vi "System Hidden Editor.vi"(6 "Channel":i32=1, 8 "Calibration in":string, 9 "Hardware in":string, 10 "Setup in":string, 11 "Editor seq info":T2 {"Steps config"."Loop Info"."unit scale" items=["Log", "Lin"]; "Steps config"."Loop Info"."unit dB ref" format="%#_6p"}) -> (1 "Step name out":string="Calibration Default", 2 "Setup out":string, 3 "Sequence channels & curves out":string[](array[string]))   [LabVIEW 2016]
uses:
  custom and Sc run Seq Sub VIs (x64).llb/editor seq info.ctl
  custom and Sc run Seq Sub VIs (x64).llb/Steps config.ctl
panel:
  in  "Wait for completion":bool
  in  "Working Directory":path
  in  "Command":string
  in  "custom setup cluster":T1={"Command Line"="", "Working Directory"=path "", "Wait for completion"=TRUE}
  in  "save":bool
  in  "cancel":bool
  # "Reminder: \nYou must edit this custom step from within a sequence for it to remember your settings."
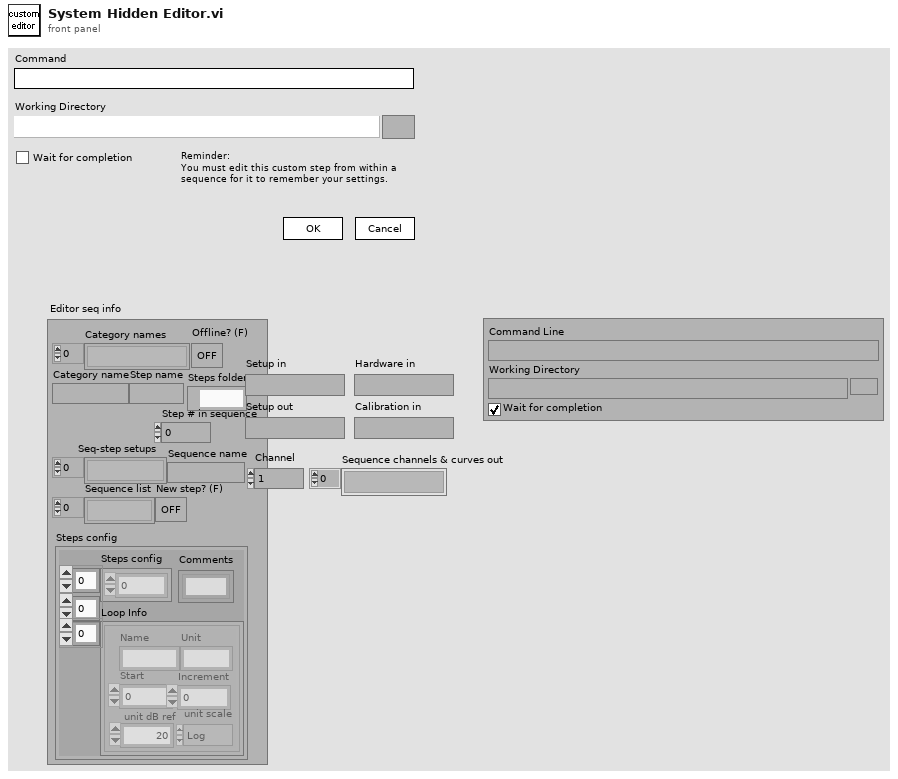
[diagram p1: front panel]
types:
  T1 = cluster{"Command Line":string, "Working Directory":path, "Wait for completion":bool}
  T2 = typedef "editor seq info.ctl" = cluster{"Category names":string[], "Category name":string, "Step name":string, "Step # in sequence":i32, "Seq-step setups":string[], "Sequence name":string, "Sequence list":string[], "New step? (F)":bool, "Steps config":T3, "Offline? (F)":bool, "Steps folder":path}
  T3 = typedef "Steps config.ctl" = cluster{"Steps config":i32[][], "Loop Info":cluster{"Name":string, "Start":dbl, "Increment":dbl, "Unit":string, "unit dB ref":dbl, "unit scale":u16}[], "Comments":string[]}
  T4 = typedef "seq step setup.ctl" = cluster{"Input Signal Channels":i32[], "Output Signal Channels":i32[], "Curves selected":string[][], "Curves generated":string[], "Step setup flat":string, "Trigger Signal Channel":i32, "Curves Generated Assumptions":cluster{"seq-setup in":string, "Relevant subset of mem list Grouping":cluster{T5[]}[]}}
  T5 = typedef "Memory List Grouping.ctl" = cluster{"item name":string, "parent":string, "Open?":bool, "Type":T6}
  T6 = typedef "Memory List Grouping - Item Type.ctl" = enum16{"item", "custom group", "auto group", "protected group"}
  T7 = typedef "waveform cluster.ctl" = cluster{"Name":string, "Waveform":cluster{"X0":dbl, "dX":dbl, "YDataRef":refnum<data-value>}, "X data":T8, "Y data":T8, "Y axis":T8, "X unit":string, "Y unit":string, "Y dB ref":dbl, "display Y":bool, "display X":bool, "Overload?":bool, "protected":bool, "Sqc history":string[], "Signal Channel ID":i32, "Plot Settings":cluster{"Color":u32, "Interpolation":u8, "Point Style":u8, "Line Style":u8, "Point Color":u32, "Line Width":u8, "Bar Plot Style":u8, "Fill To":i16}, "Test Info":string}
  T8 = typedef "Axis Unit Type.ctl" = u16
  T9 = typedef "data cluster.ctl" = cluster{"Name":string, "Curve":cluster{"x":dbl, "y":dbl, "z":dbl}[], "X data":T8, "Y data":T8, "Z data":T8, "X axis":u16, "Y axis":u16, "Z axis":u16, "X unit":string, "Y unit":string, "Z unit":string, "X dB ref":dbl, "Y dB ref":dbl, "Z dB ref":dbl, "single val":bool, "protected":bool, "display X":bool, "display Y":bool, "display Z":bool, "Plot Settings":cluster{"Color":u32, "Interpolation":u8, "Point Style":u8, "Line Style":u8, "Point Color":u32, "Line Width":u8, "Bar Plot Style":u8, "Fill To":i16}, "Test Info":string}
  T10 = typedef "result cluster.ctl" = cluster{"Name":string, "Margin":dbl, "unit":string, "Verdict":bool, "Limit":string, "Max/Min":string, "protected?":bool, "Test Info":string, "Unit type":T8}
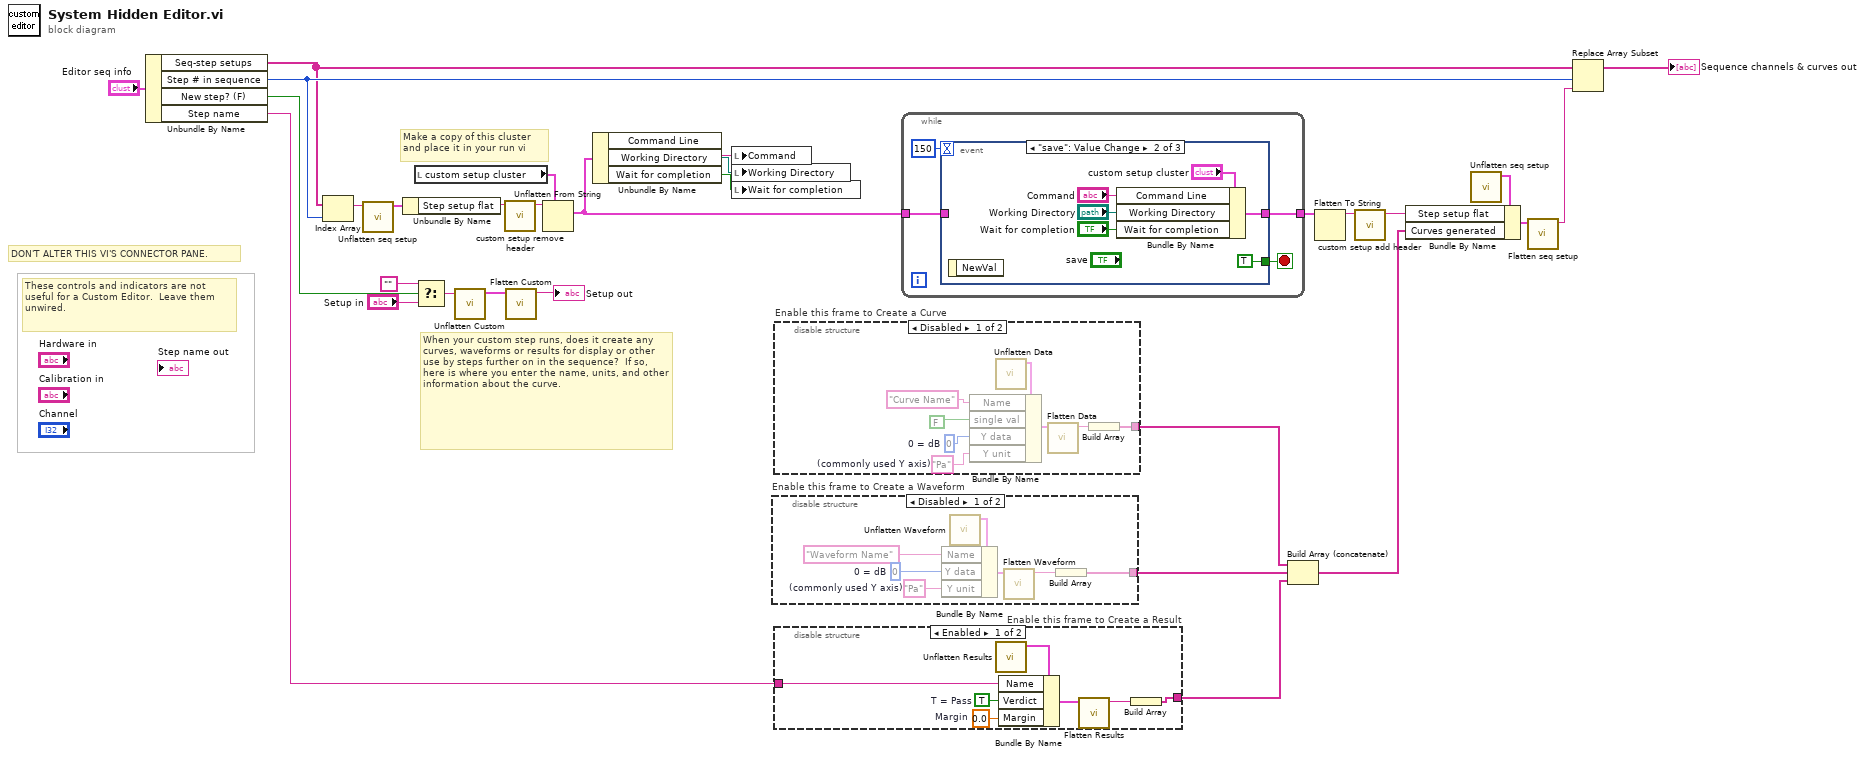
[diagram p0: block diagram]
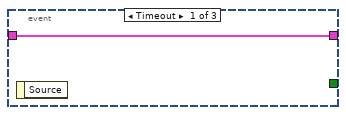
[diagram p3: hidden frame]
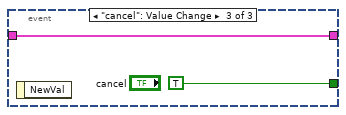
[diagram p4: hidden frame]
diagram:
  # "Make a copy of this cluster and place it in your run vi"
  # "When your custom step runs, does it create any curves, waveforms or results for display or other use by steps further on in the sequence?  If so, here is where you enter the name, units, and other information about the curve."
  # "These controls and indicators are not useful for a Custom Editor.  Leave them unwired."
  # "DON'T ALTER THIS VI'S CONNECTOR PANE."
  n1 = Unbundle By Name("Editor seq info") -> ("Seq-step setups"=w14:string[], "Step # in sequence"=w21:i32, "New step? (F)"=w25:bool, "Step name"=w8:string)
  n2 = Index Array(array=w14, index=w21) -> (element=w22:string)
  n3 = call "Unflatten seq setup.vi"("Unflatten seq setup"=w22) -> ("Sequence-specific step set-up"=w23:T4)  [unwired: 3 in, 7 out]
  n4 = Unbundle By Name(w23) -> ("Step setup flat"=w24:string)
  n5 = local read "custom setup cluster"() -> (w9:T1)
  n6 = Select(t="", s=w25, f="Setup in") -> (s? t:f=w27:string)
  n7 = call "Unflatten Custom.vi"("Unflatten Custom"=w27) -> ("Custom"=w6:cluster{"Name":string})  [unwired: 10 out]
  n8 = call "custom setup remove header.vi"("Output from 'Step setup flat' of seq-setup structure"=w24) -> ("Flattened custom step setup cluster"=w7:string)  [unwired: 10 out]
  n9 = call "Flatten Custom.vi"("Custom"=w6) -> ("Custom flattened"=→"Setup out":string)  [unwired: 10 out]
  n10 = Unflatten From String(type=w9, binary string=w7) -> (value=w4:T1)  [unwired: 1 in, 4 out]
  n11 = Unbundle By Name(w4) -> ("Command Line"=w2:string, "Working Directory"=w1:path, "Wait for completion"=w3:bool)
  n12 = local write "Command"(w2) -> ()
  n13 = local write "Working Directory"(w1) -> ()
  n14 = local write "Wait for completion"(w3) -> ()
  n15 = disable-structure "Enable this frame to Create a Waveform" shown="Disabled" {
    disable-tunnel: [w32 _] -> w11
    frame Disabled {
      w33 = "Pa"  # (commonly used Y axis)
      w36 = u16 0  # 0 = dB
      n16 = call "Unflatten Waveform.vi"() -> ("Unflattened Waveform"=w35:T7)  [unwired: 9 in, 2 out]
      n17 = Bundle By Name(cluster=w35, "Name"="Waveform Name", "Y data"=w36, "Y unit"=w33) -> (w31:T7)
      n18 = call "Flatten Waveform.vi"("Unflattened Waveform"=w31) -> ("Waveform flattened"=w37:string)  [unwired: 10 in]
      n19 = Build Array(w37) -> (w32:string[])
    }
    frame Enabled {
    }
  }
  n20 = disable-structure "Enable this frame to Create a Curve" shown="Disabled" {
    disable-tunnel: [w38 _] -> w13
    frame Disabled {
      w39 = "Pa"  # (commonly used Y axis)
      w43 = u16 0  # 0 = dB
      n21 = call "Unflatten Data.vi"() -> ("Datum"=w42:T9)  [unwired: 1 in, 10 out]
      n22 = Bundle By Name(cluster=w42, "Name"="Curve Name", "single val"=FALSE, "Y data"=w43, "Y unit"=w39) -> (w40:T9)
      n23 = call "Flatten Data.vi"("Datum"=w40) -> ("Data flattened"=w45:string)  [unwired: 10 out]
      n24 = Build Array(w45) -> (w38:string[])
    }
    frame Enabled {
    }
  }
  n25 = disable-structure "Enable this frame to Create a Result" shown="Enabled" {
    disable-tunnel: [w50 _] -> w12
    disable-tunnel: w8 -> [w46 _]
    frame Enabled {
      w47 = 0.0  # Margin
      w48 = TRUE  # T = Pass
      n26 = call "Unflatten Results.vi"() -> ("Result"=w51:T10)  [unwired: 9 in, 2 out]
      n27 = Bundle By Name(cluster=w51, "Name"=w46, "Verdict"=w48, "Margin"=w47) -> (w49:T10)
      n28 = call "Flatten Results.vi"("Result"=w49) -> ("Result flattened"=w52:string)  [unwired: 10 in]
      n29 = Build Array(w52) -> (w50:string[])
    }
    frame Disabled {
    }
  }
  n30 = while {
    tunnel: [w54] -> w15
    tunnel: w4 -> [w53]
    stop <- w55 stop-if-true
    n31 = event shown="[1] \"save\": Value Change" {
      selector: _ -> [_ _ _]
      dyn-events: _ -> [_ _ _]
      timeout: 150 -> [_ _ _]
      tunnel: [_ TRUE TRUE] -> w55
      tunnel: [w57 w61 w64] -> w54
      tunnel: w53 -> [w57 _ w64]
      event Timeout {
        n32 = event-data() -> ()  [unwired: 1 in, 1 out]
      }
      event "save": Value Change {
        n33 = event-data() -> ()  [unwired: 1 in, 1 out]
        n34 = Bundle By Name(cluster="custom setup cluster", "Command Line"="Command", "Working Directory"="Working Directory", "Wait for completion"="Wait for completion") -> (w61:T1)
      }
      event "cancel": Value Change {
        n35 = event-data() -> ()  [unwired: 1 in, 1 out]
      }
    }
  }
  n36 = Build Array (concatenate)(w13, w11, w12) -> (w10:string[])
  n37 = Flatten To String(anything=w15) -> (data string=w17:string)  [unwired: 2 in, 3 out]
  n38 = call "custom setup add header.vi"("Flattened custom step setup cluster"=w17) -> ("Input to 'Step setup flat' of seq-setup structure"=w5:string)  [unwired: 1 in, 9 out]
  n39 = call "Unflatten seq setup.vi"() -> ("Sequence-specific step set-up"=w20:T4)  [unwired: 4 in, 7 out]
  n40 = Bundle By Name(cluster=w20, "Step setup flat"=w5, "Curves generated"=w10) -> (w19:T4)
  n41 = call "Flatten seq setup.vi"("Sequence-specific step set-up"=w19) -> ("Seq setup flattened"=w18:string)  [unwired: 10 out]
  n42 = Replace Array Subset(array=w14, new element=w18, index=w21) -> (→"Sequence channels & curves out":string[])
